vi "testTwoServersReportConnStatusMultipleTimes.vi"(8 "error in":errorcluster) -> (0 "error out":errorcluster)   [LabVIEW 2018]
uses:
  src/FactoryTcpServer/FactoryTcpServer.lvclass
  <vilib>/addons/_JKI Toolkits/Caraya/classes/Assert/Assert Equal Value_Variant.vi
  src/TcpServer/TcpServer.lvclass
  <vilib>/addons/_JKI Toolkits/Caraya/classes/Test/Test.lvclass
  <vilib>/addons/_JKI Toolkits/Caraya/classes/Assert/Assert.lvclass
panel:
  out "Run Server B error":errorcluster
  out "Run Server A error":errorcluster
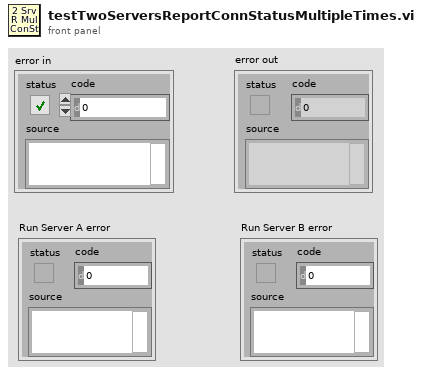
[diagram p1: front panel]
types:
  T1 = cluster{"CmdRead":refnum<user-event>, "EvtRead":refnum<user-event>, "GenRead":refnum<user-event>}
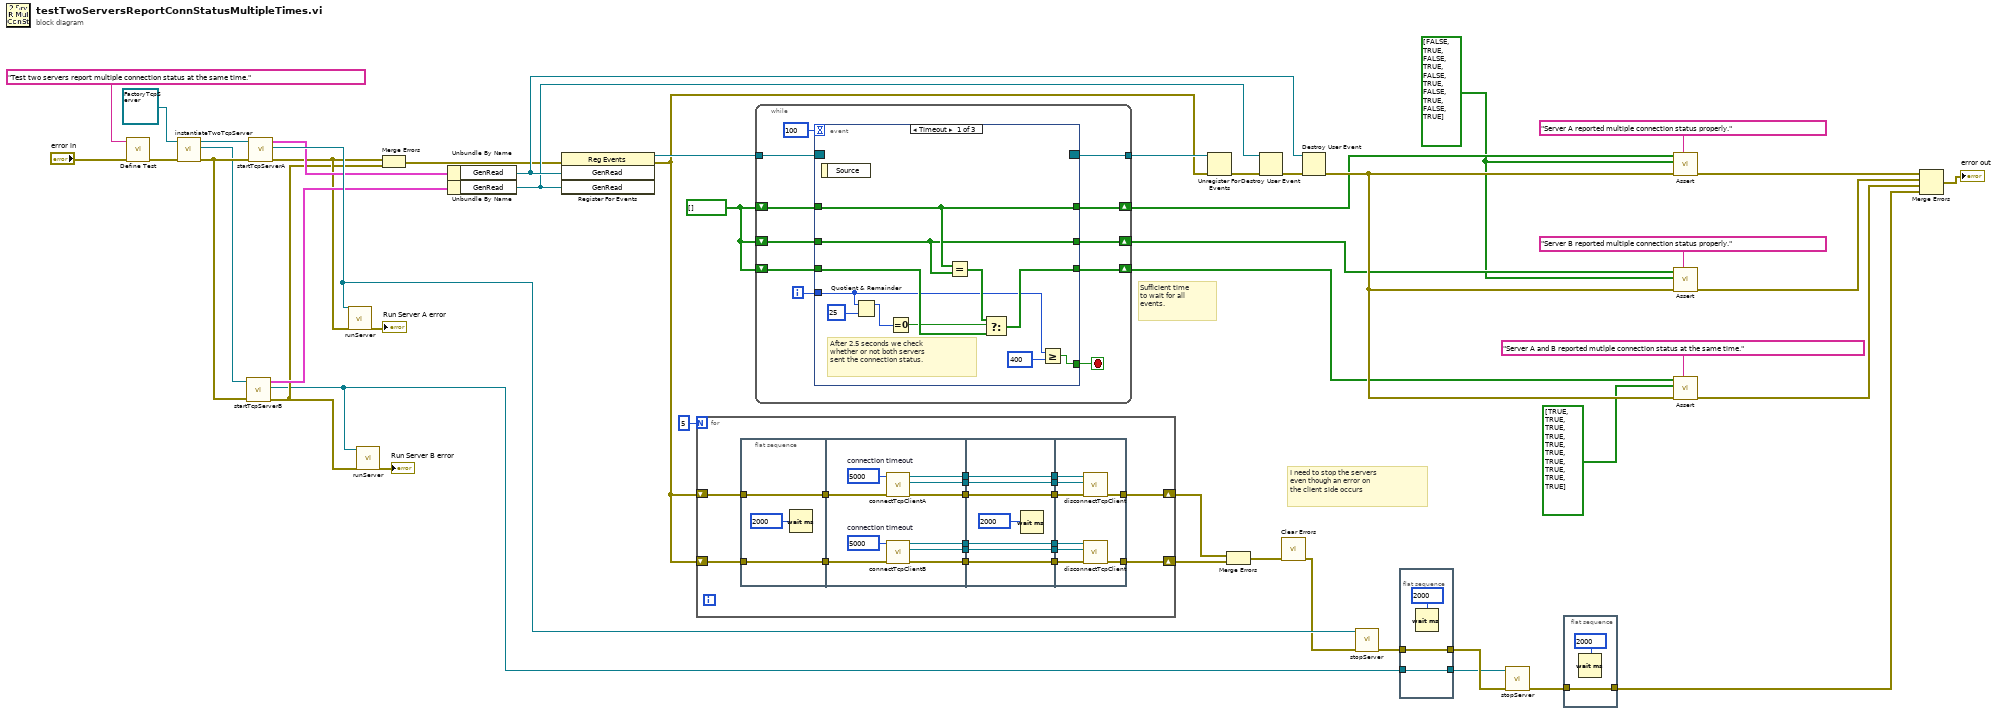
[diagram p0: block diagram]
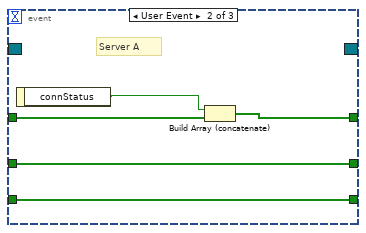
[diagram p2: hidden frame]
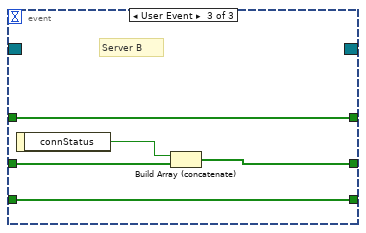
[diagram p3: hidden frame]
diagram:
  w4 = bool[] [FALSE, TRUE, FALSE, TRUE, FALSE, TRUE, FALSE, TRUE, FALSE, TRUE]
  w5 = bool[] []
  # "Sufficient time \nto wait for all \nevents."
  # "I need to stop the servers \neven though an error on \nthe client side occurs"
  n1 = call <vilib>:"Define Test.vi"("error in (no error)"="error in", "Label (VI Title)"="Test two servers report multiple connection status at the same time.") -> ("error out"=w42:errorcluster)  [unwired: 9 in]
  n2 = call "instantiateTwoTcpServer.vi"("error in (no error)"=w42, "FactoryTcpServer in"=refnum<class "FactoryTcpServer.lvclass"> refnum) -> ("error out"=w18:errorcluster, "TcpServer 2 out"=w15:refnum<class "TcpServer.lvclass">, "TcpServer 1 out"=w16:refnum<class "TcpServer.lvclass">)  [unwired: 6 in, 1 out]
  n3 = call "startTcpServerB.vi"("error in (no error)"=w18, "TcpServer.lvclass"=w15) -> ("error out"=w19:errorcluster, "TcpServer out"=w10:refnum<class "TcpServer.lvclass">, "UserEvents"=w39:T1)  [unwired: 7 in]
  n4 = call "startTcpServerA.vi"("error in (no error)"=w18, "TcpServer.lvclass"=w16) -> ("error out"=w30:errorcluster, "TcpServer out"=w41:refnum<class "TcpServer.lvclass">, "UserEvents"=w40:T1)  [unwired: 7 in]
  n5 = call "runServer.vi"("error in (no error)"=w30, "TcpServer in"=w41) -> ("error out (no error)"=→"Run Server A error":errorcluster)  [unwired: 8 in, 1 out]
  n6 = call "runServer.vi"("error in (no error)"=w19, "TcpServer in"=w10) -> ("error out (no error)"=→"Run Server B error":errorcluster)  [unwired: 8 in, 1 out]
  n7 = Merge Errors(w30, w19) -> (w20:errorcluster)
  n8 = Unbundle By Name(w40) -> ("GenRead"=w33:refnum<user-event>)
  n9 = Unbundle By Name(w39) -> ("GenRead"=w26:refnum<user-event>)
  n10 = register-events(error in=w20, w33, w26) -> (reference out=w38:refnum<event-registration>, error out=w1:errorcluster)  [unwired: 1 in]
  n11 = for {
    N: 5 -> [_]
    shift-right: [w51] -> w36
    shift-left: w1 -> [w49]
    shift-right: [w50] -> w35
    shift-left: w1 -> [w48]
    n12 = flat-sequence {
      tunnel: [w67] -> w65
      tunnel: w49 -> [w67]
      tunnel: [w66] -> w64
      tunnel: w48 -> [w66]
      tunnel: [w78] -> w63
      tunnel: [w77] -> w62
      tunnel: [w76] -> w61
      tunnel: [w75] -> w60
      tunnel: [w74] -> w59
      tunnel: [w73] -> w58
      tunnel: w65 -> [w72]
      tunnel: w64 -> [w71]
      tunnel: [w84] -> w57
      tunnel: w63 -> [w84]
      tunnel: [w83] -> w56
      tunnel: w62 -> [w83]
      tunnel: [w82] -> w55
      tunnel: w61 -> [w82]
      tunnel: [w81] -> w54
      tunnel: w60 -> [w81]
      tunnel: [w80] -> w53
      tunnel: w59 -> [w80]
      tunnel: [w79] -> w52
      tunnel: w58 -> [w79]
      tunnel: w57 -> [w93]
      tunnel: w56 -> [w92]
      tunnel: w55 -> [w91]
      tunnel: w54 -> [w90]
      tunnel: w53 -> [w89]
      tunnel: w52 -> [w88]
      tunnel: [w87] -> w51
      tunnel: [w86] -> w50
      frame #0 {
        n13 = Wait (ms)(milliseconds to wait=u32 2000) -> ()  [unwired: 1 out]
      }
      frame #1 {
        w69 = 5000  # connection timeout
        w70 = 5000  # connection timeout
        n14 = call "connectTcpClientA.vi"("error in (no error)"=w72, "connection timeout (ms)"=w70) -> ("error out"=w76:errorcluster, "tel connection ID A out"=w77:refnum<k5>, "cmd connection ID A out"=w78:refnum<k5>)  [unwired: 7 in]
        n15 = call "connectTcpClientB.vi"("error in (no error)"=w71, "connection timeout (ms)"=w69) -> ("error out"=w73:errorcluster, "tel connection ID B out"=w74:refnum<k5>, "cmd connection ID B out"=w75:refnum<k5>)  [unwired: 7 in]
      }
      frame #2 {
        n16 = Wait (ms)(milliseconds to wait=u32 2000) -> ()  [unwired: 1 out]
      }
      frame #3 {
        n17 = call "disconnectTcpClient.vi"("error in (no error)"=w91, "tel connection ID in"=w92, "cmd connection ID in"=w93) -> ("error out"=w87:errorcluster)  [unwired: 8 in]
        n18 = call "disconnectTcpClient.vi"("error in (no error)"=w88, "tel connection ID in"=w89, "cmd connection ID in"=w90) -> ("error out"=w86:errorcluster)  [unwired: 8 in]
      }
    }
  }
  n19 = while {
    tunnel: [w104] -> w37
    tunnel: w38 -> [w102]
    shift-right: [w95] -> w3
    shift-left: w5 -> [w101]
    shift-right: [w98] -> w7
    shift-left: w5 -> [w99]
    shift-right: [w97] -> w6
    shift-left: w5 -> [w96]
    i -> [w100]
    stop <- w94 stop-if-true
    # "Event Structure for TCP server A"
    n20 = event shown="[0] Timeout" {
      selector: w102 -> [_ _ _]
      dyn-events: [_ _ _] -> w104
      timeout: 100 -> [_ _ _]
      tunnel: [w109 w116 w121] -> w95
      tunnel: w101 -> [w110 w116 w121]
      tunnel: w100 -> [w107 _ _]
      tunnel: w99 -> [w115 w120 w125]
      tunnel: [w115 w118 w125] -> w98
      tunnel: [w114 w117 w124] -> w97
      tunnel: w96 -> [w114 w117 w123]
      tunnel: [w106 _ _] -> w94
      event Timeout {
        # "After 2.5 seconds we check\nwhether or not both servers\nsent the connection status."
        n21 = event-data() -> ()  [unwired: 1 in, 1 out]
        n22 = Quotient & Remainder(x=w107, y=25) -> (x-y*floor(x/y)=w112:i32)  [unwired: 1 out]
        n23 = Equal To 0?(x=w112) -> (x = 0?=w108:bool)
        n24 = Equal?(x=w115, y=w114) -> (x = y?=w111:bool[])
        n25 = Select(t=w111, s=w108, f=w110) -> (s? t:f=w109:bool[])
        n26 = Greater Or Equal?(x=w107, y=400) -> (x >= y?=w106:bool)
      }
      event User Event {
        # "Server A"
        n27 = event-data() -> ("connStatus"=w119:bool)  [unwired: 1 in]
        n28 = Build Array (concatenate)(w119, w120) -> (w118:bool[])
      }
      event User Event {
        # "Server B"
        n29 = event-data() -> ("connStatus"=w122:bool)  [unwired: 1 in]
        n30 = Build Array (concatenate)(w122, w123) -> (w124:bool[])
      }
    }
  }
  n31 = Unregister For Events(event registration refnum=w37, error in=w1) -> (error out=w28:errorcluster)
  n32 = Merge Errors(w36, w35) -> (w34:errorcluster)
  n33 = Destroy User Event(user event=w26, error in=w28) -> (error out=w27:errorcluster)
  n34 = call <vilib>:"Clear Errors.vi"("error in (no error)"=w34) -> ("error out"=w13:errorcluster)  [unwired: 5 in, 1 out]
  n35 = Destroy User Event(user event=w33, error in=w27) -> (error out=w14:errorcluster)
  n36 = call "stopServer.vi"("error in (no error)"=w13, "tcpServer in"=w41) -> ("error out"=w11:errorcluster)  [unwired: 8 in, 1 out]
  n37 = flat-sequence {
    tunnel: [w127] -> w12
    tunnel: w11 -> [w127]
    tunnel: w10 -> [w126]
    tunnel: [w126] -> w9
    frame #0 {
      n38 = Wait (ms)(milliseconds to wait=u32 2000) -> ()  [unwired: 1 out]
    }
  }
  n39 = call "stopServer.vi"("error in (no error)"=w12, "tcpServer in"=w9) -> ("error out"=w44:errorcluster)  [unwired: 8 in, 1 out]
  n40 = flat-sequence {
    tunnel: w44 -> [w129]
    tunnel: [w129] -> w23
    frame #0 {
      n41 = Wait (ms)(milliseconds to wait=u32 2000) -> ()  [unwired: 1 out]
    }
  }
  n42 = call-poly <vilib>:"Assert.vi"("Label"="Server A reported multiple connection status properly.", "error in (no error)"=w14, "Y"=w4, "X"=w7) -> ("error out"=w29:errorcluster)  [unwired: 7 in]
  n43 = call-poly <vilib>:"Assert.vi"("Label"="Server B reported multiple connection status properly.", "error in (no error)"=w14, "Y"=w4, "X"=w6) -> ("error out"=w22:errorcluster)  [unwired: 7 in]
  n44 = call-poly <vilib>:"Assert.vi"("Label"="Server A and B reported mutlple connection status at the same time.", "error in (no error)"=w14, "Y"=bool[] [TRUE, TRUE, TRUE, TRUE, TRUE, TRUE, TRUE, TRUE, TRUE, TRUE], "X"=w3) -> ("error out"=w21:errorcluster)  [unwired: 7 in]
  n45 = Merge Errors(w29, w22, w21, w23) -> (→"error out":errorcluster)
